vi "connect_database.vi"(8 "error in (no error)":errorcluster, 10 "Database Path":path, 11 "object in":refnum<class "SQLiteConnection.lvclass">) -> (0 "error out":errorcluster, 3 "object out":refnum<class "SQLiteConnection.lvclass">)   [LabVIEW 2019, in "SQLiteConnection.lvclass"]
uses:
  SQLiteConnection.lvclass
  SQLiteConnection.lvclass/SQLiteConnection.ctl
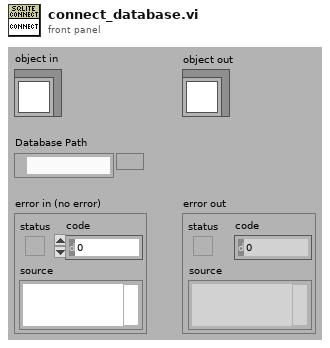
[diagram p1: front panel]
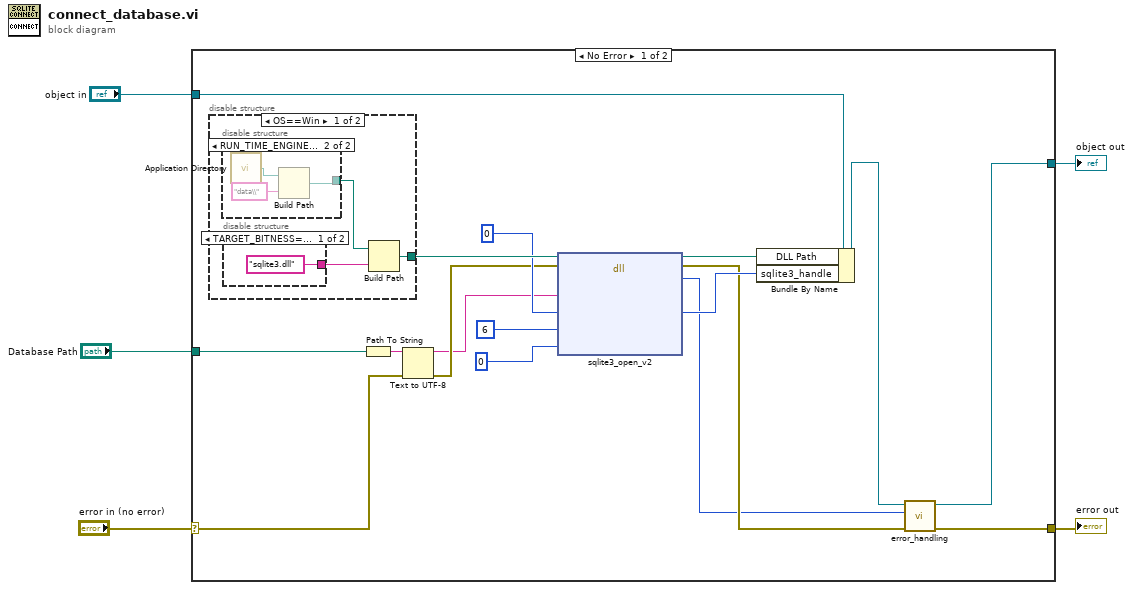
[diagram p0: block diagram]
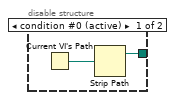
[diagram p2: hidden frame]
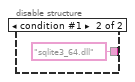
[diagram p3: hidden frame]
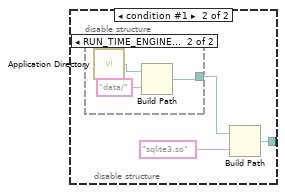
[diagram p4: hidden frame]
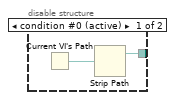
[diagram p5: hidden frame]
diagram:
  n1 = case shown="No Error" "error in (no error)" {
    selector: "error in (no error)" -> [w8 w42]
    tunnel: [w17 w42] -> w4
    tunnel: [w14 w41] -> w2
    tunnel: "object in" -> [w22 w41]
    tunnel: "Database Path" -> [w10 _]
    frame No Error {
      n2 = disable-structure shown="OS==Win" {
        disable-tunnel: [w24 w34] -> w21
        frame condition #0 (active) {
          n3 = disable-structure shown="RUN_TIME_ENGINE==True" {
            disable-tunnel: [w26 w29] -> w23
            frame condition #0 (active) {
              n4 = Current VI's Path() -> (path=w27:path)
              n5 = Strip Path(path=w27) -> (stripped path=w26:path)  [unwired: 1 out]
            }
            frame condition #1 {
              n6 = call <vilib>:"Application Directory.vi"() -> ("Application Directory"=w30:path)
              n7 = Build Path(base path=w30, name or relative path="data\\") -> (appended path=w29:path)
            }
          }
          n8 = disable-structure shown="TARGET_BITNESS==32, 扁夯" {
            disable-tunnel: ["sqlite3.dll" ("name or relative path") "sqlite3_64.dll" ("name or relative path")] -> w25
            frame condition #0 (active) {
            }
            frame condition #1 {
            }
          }
          n9 = Build Path(base path=w23, name or relative path=w25) -> (appended path=w24:path)
        }
        frame condition #1 {
          n10 = disable-structure shown="RUN_TIME_ENGINE==True" {
            disable-tunnel: [w36 w39] -> w33
            frame condition #0 (active) {
              n11 = Current VI's Path() -> (path=w37:path)
              n12 = Strip Path(path=w37) -> (stripped path=w36:path)  [unwired: 1 out]
            }
            frame condition #1 {
              n13 = call <vilib>:"Application Directory.vi"() -> ("Application Directory"=w40:path)
              n14 = Build Path(base path=w40, name or relative path="data/") -> (appended path=w39:path)
            }
          }
          n15 = Build Path(base path=w33, name or relative path="sqlite3.so") -> (appended path=w34:path)
        }
      }
      n16 = Path To String(path=w10) -> (string=w7:string)
      n17 = Text to UTF-8(8:w8, 11:w7) -> (0:w9:errorcluster, 3:w6:string)  [unwired: 1 in]
      n18 = dll-call lib="D:/Users/mcarl/Documents/LabVIEW Projects/OW-PIKO/OW-PIKO Software/sqlite3.dll" fn="sqlite3_open_v2"(path in=w21, error in=w9, "path"=w6, "sqlitehandle"=u64 0, "flags"=6, "unused"=u64 0) -> (path out=w19:path, error out=w18:errorcluster, "return type"=w16:i32, "sqlitehandle"=w20:u64)  [unwired: 4 in]
      n19 = Bundle By Name(cluster=w22, "DLL Path"=w19, "sqlite3_handle"=w20) -> (w15:refnum<class "SQLiteConnection.lvclass">)
      n20 = call "error_handling.vi"("error in (no error)"=w18, "error handle"=w16, "object in"=w15) -> ("error out"=w17:errorcluster, "object out"=w14:refnum<class "SQLiteConnection.lvclass">)  [unwired: 7 in]
    }
    frame Error {
    }
  }
  "error out" <- w4
  "object out" <- w2
